vi "Test Iterate over Array Add.vi"() -> ()   [LabVIEW 2021]
uses:
  Source/Variable/Double Float Array/Double Float Array 1D.lvclass
  C:/Users/Tim/Documents/LabVIEW/2021/Data Classes/Source/Element/Vector Parent/Vector Parent.lvclass
  Source/Element/Vector Parent/Vector Parent.lvclass/Vector Parent.ctl
  Source/Element/Vector Parent/Properties/Write Size.vi
panel:
  in  "stop":bool
  in  "Index":i32=50
  out "Valid Index":bool
  out "Numeric":dbl
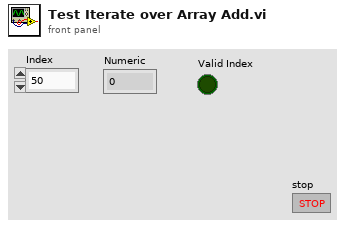
[diagram p1: front panel]
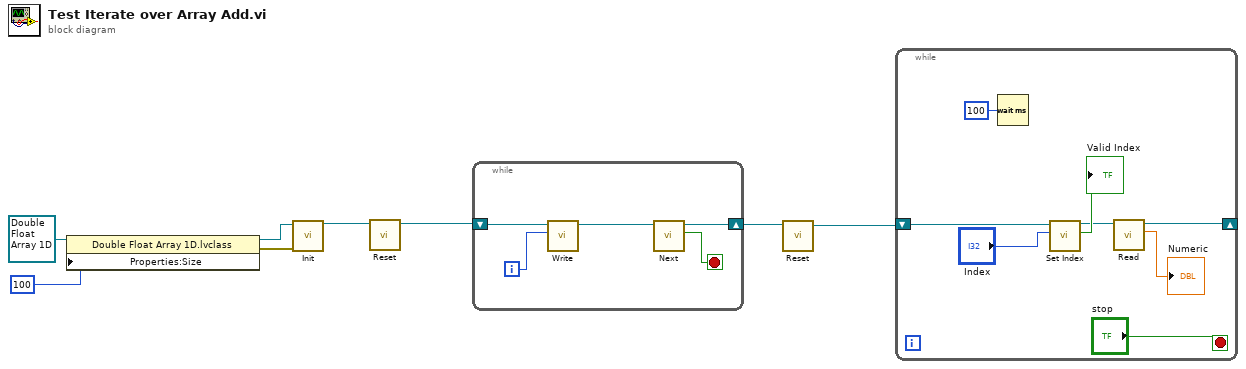
[diagram p0: block diagram]
diagram:
  n1 = property class="Double Float Array 1D.lvclass"(reference=refnum<class "Double Float Array 1D.lvclass"> refnum ("Variable.lvlib:Numeric Array.lvclass"), "Properties:Size"=100) -> (reference out=w6:refnum<class "Double Float Array 1D.lvclass">, error out=w8:errorcluster)  [unwired: 1 in]
  n2 = call-dynamic "Init.vi"("error in (no error)"=w8, "Data in"=w6) -> ("Data out"=w4:refnum<class "Double Float Array 1D.lvclass">)  [unwired: 8 in, 1 out]
  n3 = call-dynamic "Reset.vi"("Vector in"=w4) -> ("Vector out"=w3:refnum<class "Double Float Array 1D.lvclass">)  [unwired: 9 in, 1 out]
  n4 = while {
    shift-right: [w9] -> w2
    shift-left: w3 -> [w11]
    i -> [w12]
    stop <- w13 stop-if-true
    n5 = call-dynamic "Write.vi"("Numeric"=w12, "Numeric Array in"=w11) -> ("Numeric Array out"=w10:refnum<class "Double Float Array 1D.lvclass">)  [unwired: 8 in, 1 out]
    n6 = call-dynamic "Next.vi"("Vector in"=w10) -> ("Last?"=w13:bool, "Vector out"=w9:refnum<class "Double Float Array 1D.lvclass">)  [unwired: 8 in, 1 out]
  }
  n7 = call-dynamic "Reset.vi"("Vector in"=w2) -> ("Vector out"=w1:refnum<class "Double Float Array 1D.lvclass">)  [unwired: 9 in, 1 out]
  n8 = while {
    shift-right: [w15] -> _
    shift-left: w1 -> [w21]
    stop <- "stop" stop-if-true
    n9 = Wait (ms)(milliseconds to wait=u32 100) -> ()  [unwired: 1 out]
    n10 = call-dynamic "Set Index.vi"("Index"="Index", "Array in"=w21) -> ("In Range?"=→"Valid Index":bool, "Array out"=w14:refnum<class "Double Float Array 1D.lvclass">)  [unwired: 7 in, 1 out]
    n11 = call-dynamic "Read.vi"("Numeric Array in"=w14) -> ("Numeric"=→"Numeric":dbl, "Numeric Array out"=w15:refnum<class "Double Float Array 1D.lvclass">)  [unwired: 8 in, 1 out]
  }
